vi "proiectu fara drona_with_phone.vi"() -> ()   [LabVIEW 2015]
uses:
  <vilib>/vision/driver/NI_Vision_Acquisition_Software.lvlib
  <vilib>/userdefined/High Color/IMAQdx.ctl
panel:
  out "Grabbing images":bool
  in  "Tab Control":T1(tab)
  in  "Grab picture":bool
  out "Number of photos":i32
  in  "Stop grabbing":bool
  out "Please select your destination":T2(plugin-control)
  out "START LOCATION":T2(plugin-control)
  out "CAR PATH":T2(plugin-control)
  out "Elapsed time":dbl
  out "Color segmentation":bool
  out "Started creating image from matrix":bool
  in  "?":bool
  out "Computing Path for the car":bool
  out "Finding START/STOP":bool
  out "Started stitching":bool
  # "Please wait while the images are processed and stitched together!"
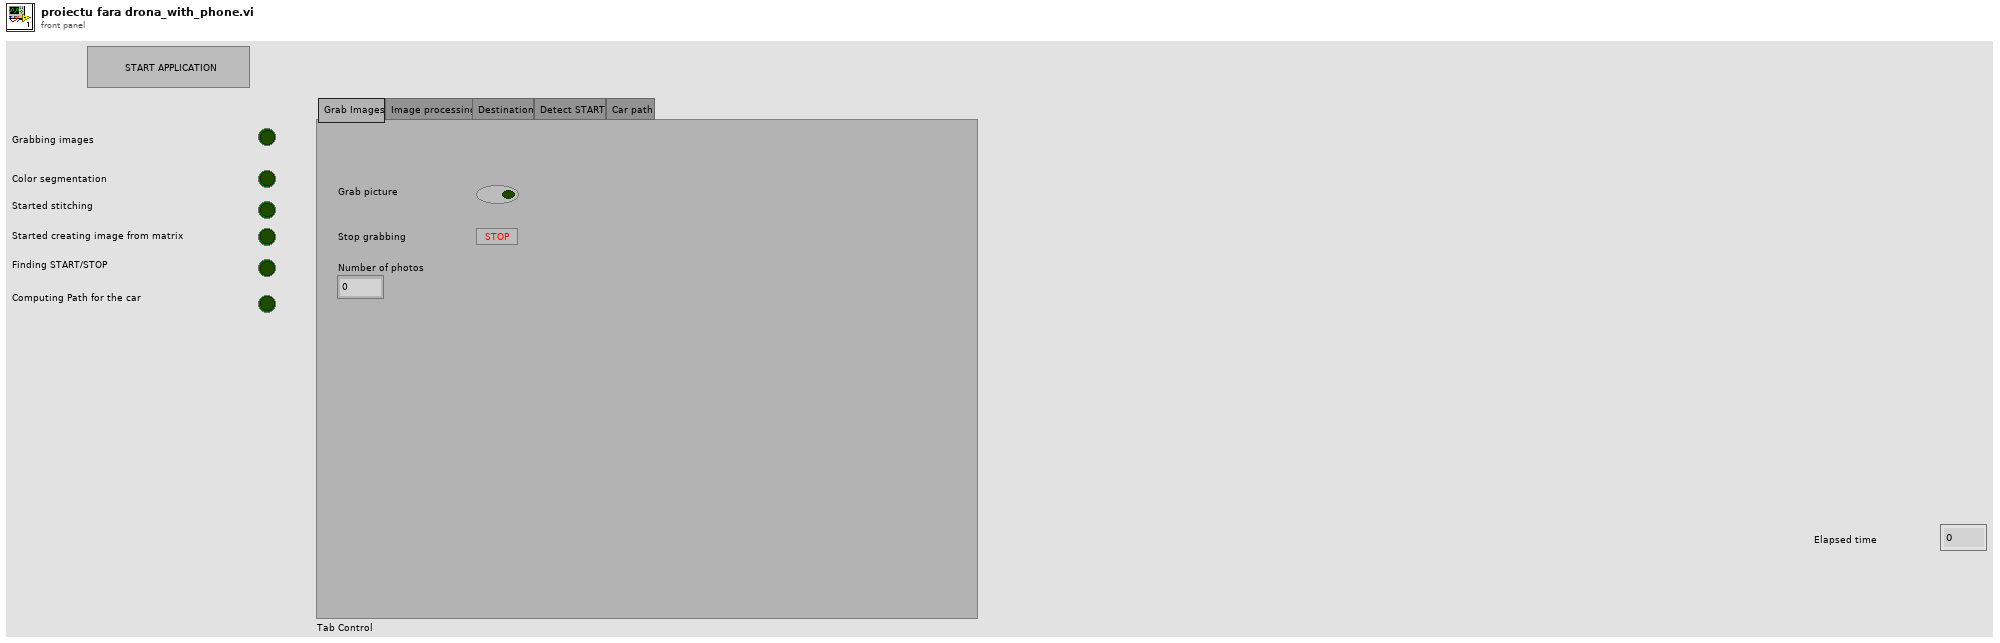
[diagram p1: front panel]
types:
  T1 = enum32{"Grab Images", "Image processing", "Destination", "Detect START", "Car path"}
  T2 = typedef "IMAQ Image.ctl" = refnum<image>
  T3 = typedef "IMAQdx.ctl" = refnum<k21>
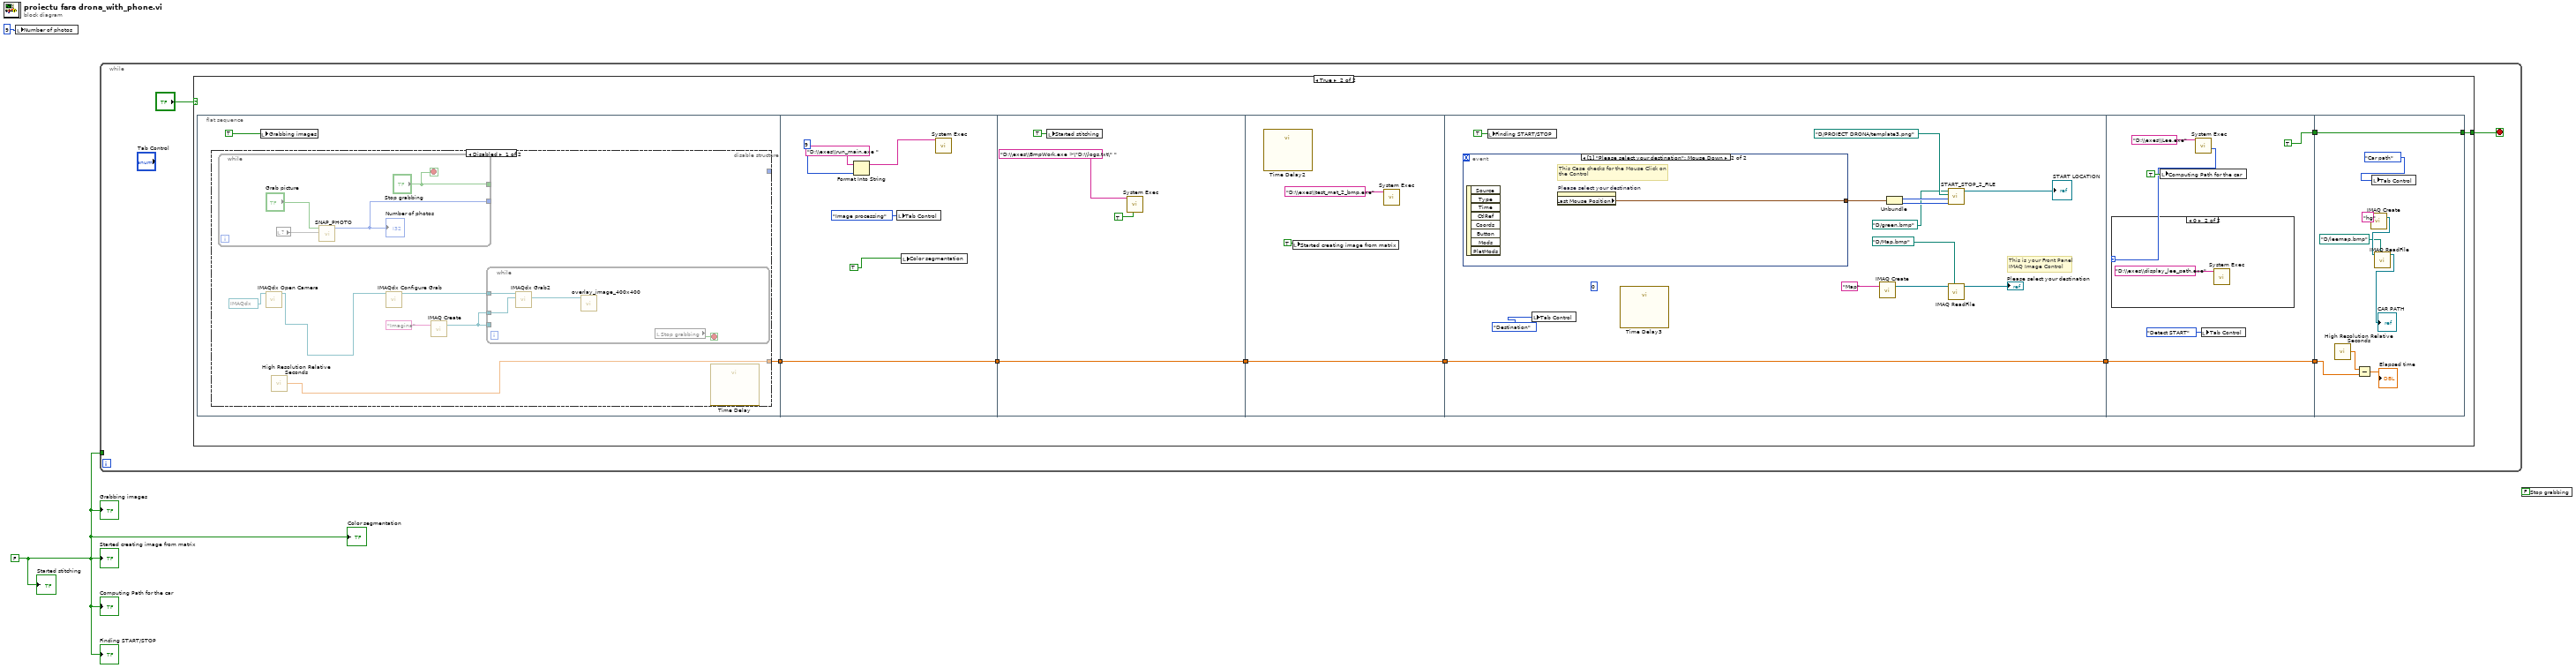
[diagram p0: block diagram]
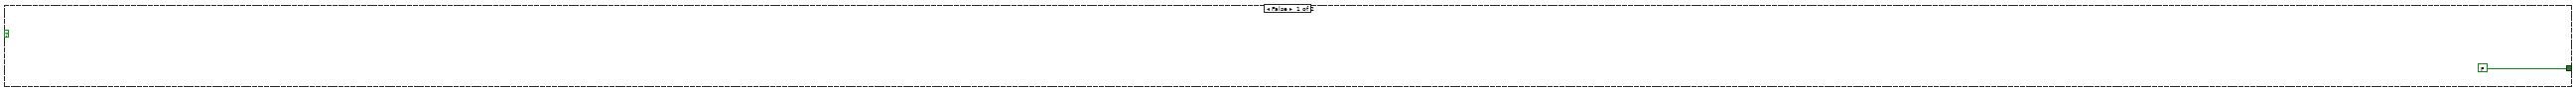
[diagram p2: hidden frame]
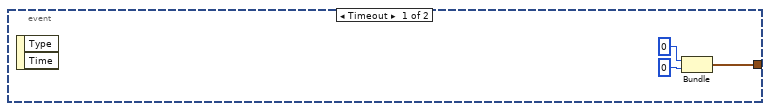
[diagram p4: hidden frame]
diagram:
  w1 = FALSE
  n1 = local write "Number of photos"(9 ("Number of photos")) -> ()
  n2 = while {
    tunnel: w1 -> [_]
    stop <- w4 stop-if-true
    n3 = case shown="True" "?" {
      tunnel: [FALSE w14] -> w4
      frame False {
      }
      frame True {
        n4 = flat-sequence {
          tunnel: [w15] -> w7
          tunnel: [w37] -> w8
          tunnel: w7 -> [w37]
          tunnel: [w40] -> w9
          tunnel: w8 -> [w40]
          tunnel: [w43] -> w10
          tunnel: w9 -> [w43]
          tunnel: [w48] -> w11
          tunnel: w10 -> [w48]
          tunnel: [TRUE] -> w13
          tunnel: [w64] -> w12
          tunnel: w11 -> [w64]
          tunnel: [w78] -> w14
          tunnel: w13 -> [w78]
          tunnel: w12 -> [w71]
          frame #0 {
            n5 = disable-structure shown="Disabled" {
              disable-tunnel: [w18 _] -> w15
              disable-tunnel: _ -> [w17 _]
              frame Disabled {
                n6 = while {
                  tunnel: ["Stop grabbing"] -> _
                  tunnel: [w29] -> _
                  stop <- "Stop grabbing" stop-if-true
                  n7 = local read item#-1() -> (w31)
                  n8 = call "SNAP_PHOTO.vi"("Image"=w31, "Boolean"="Grab picture") -> ("Numeric 2"=w29:i32)  [unwired: 9 in]
                  "Number of photos" <- w29
                }
                n9 = call <vilib>:"IMAQdx Open Camera.vi"("Session In"=T3 "cam2") -> ("Session Out"=w19:T3)  [unwired: 9 in, 1 out]
                n10 = call <vilib>:"High Resolution Relative Seconds.vi"() -> ("relative seconds"=w18:dbl)
                n11 = call <vilib>:"IMAQdx Configure Grab.vi"("Session In"=w19) -> ("Session Out"=w21:T3)  [unwired: 9 in, 1 out]
                n12 = call "IMAQ Create"("Image Name"="Imagina") -> ("New Image"=w22:T2)  [unwired: 4 in, 1 out]
                n13 = while {
                  tunnel: w22 -> [_]
                  tunnel: w22 -> [w28]
                  tunnel: w21 -> [w27]
                  stop <- w26 stop-if-true
                  n14 = call <vilib>:"IMAQdx Grab2.vi"("Image In"=w28, "Session In"=w27) -> ("Image Out"=w25:T2)  [unwired: 6 in, 3 out]
                  n15 = call "overlay_image_400x400.vi"("Image 2"=w25) -> ("Image"=w24:T2)  [unwired: 10 in]
                  n16 = local read "Stop grabbing"() -> (w26:bool)
                }
                n17 = call "Time Delay"() -> ()  [unwired: 11 in, 1 out]
              }
              frame Enabled {
              }
            }
            n18 = local write "Grabbing images"(TRUE) -> ()
          }
          frame #1 {
            n19 = Format Into String(initial string="D:\\exes\\run_main.exe ", 9) -> (resulting string=w35:string)  [unwired: 2 in, 1 out]
            n20 = local write "Tab Control"(T1."Image processing" ("Tab Control")) -> ()
            n21 = local write "Color segmentation"(TRUE) -> ()
            n22 = call <vilib>:"System Exec.vi"("command line"=w35) -> ()  [unwired: 7 in, 4 out]
          }
          frame #2 {
            n23 = local write "Started stitching"(TRUE) -> ()
            n24 = call <vilib>:"System Exec.vi"("run minimized? (F)"=TRUE, "command line"="D:\\exes\\BmpWork.exe >\"D:\\logs.txt\" ") -> ()  [unwired: 6 in, 4 out]
          }
          frame #3 {
            n25 = call "Time Delay2"() -> ()  [unwired: 11 in, 1 out]
            n26 = local write "Started creating image from matrix"(TRUE) -> ()
            n27 = call <vilib>:"System Exec.vi"("command line"="D:\\exes\\test_mat_2_bmp.exe") -> ()  [unwired: 7 in, 4 out]
          }
          frame #4 {
            (unwired) 0 ("index")
            # "This is your Front Panel\nIMAQ Image Control"
            n28 = event shown="[1] \"Please select your destination\": Mouse Down" {
              selector: _ -> [_ _]
              dyn-events: _ -> [_ _]
              timeout: _ -> [_ _]
              tunnel: [w59 w62] -> w49
              event Timeout {
                n29 = event-data() -> ()  [unwired: 3 out]
                n30 = Bundle(0, 0) -> (w59:cluster{i32, i32})  [unwired: 1 in]
              }
              event "Please select your destination": Mouse Down {
                # "This Case checks for the Mouse Click on\nthe Control"
                n31 = event-data() -> ()  [unwired: 9 out]
                n32 = property on="Please select your destination" class="ImageControl"() -> ("Last Mouse Position"=w62:cluster{"X":i32, "Y":i32})  [unwired: 2 in, 2 out]
              }
            }
            n33 = local write "Finding START/STOP"(TRUE) -> ()
            n34 = local write "Tab Control"(T1."Destination" ("Tab Control")) -> ()
            n35 = call "Time Delay3"() -> ()  [unwired: 11 in, 1 out]
            n36 = call "IMAQ Create"("Image Name"="Map") -> ("New Image"=w55:T2)  [unwired: 4 in, 1 out]
            n37 = Unbundle(w49) -> ("X"=w51:i32, "Y"=w50:i32)
            n38 = call "START_STOP_2_FILE.vi"("stop_y"=w50, "stop_x"=w51, "Template"=path "D:/PROIECT DRONA/template3.png" ("Path to template"), "MAP"=path "D:/green.bmp") -> ("Image"=→"START LOCATION":T2)  [unwired: 7 in]
            n39 = call "IMAQ ReadFile"("File Path"=path "D:/Map.bmp" ("Fisierul Text"), "Image"=w55) -> ("Image Out"=→"Please select your destination":T2)  [unwired: 5 in, 4 out]
          }
          frame #5 {
            n40 = local write "Computing Path for the car"(TRUE) -> ()
            n41 = call <vilib>:"System Exec.vi"("command line"="D:\\exes\\Lee.exe") -> ("return code"=w65:i32)  [unwired: 7 in, 3 out]
            n42 = case shown="0" w65 {
              frame Default {
              }
              frame 0 {
                n43 = call <vilib>:"System Exec.vi"("command line"="D:\\exes\\display_lee_path.exe") -> ()  [unwired: 7 in, 4 out]
              }
            }
            n44 = local write "Tab Control"(T1."Detect START" ("Tab Control")) -> ()
          }
          frame #6 {
            n45 = call <vilib>:"High Resolution Relative Seconds.vi"() -> ("relative seconds"=w72:dbl)
            n46 = Subtract(x=w72, y=w71) -> (x-y=→"Elapsed time":dbl)
            n47 = call "IMAQ Create"("Image Name"="hg") -> ("New Image"=w76:T2)  [unwired: 4 in, 1 out]
            n48 = local write "Tab Control"(T1."Car path" ("Tab Control")) -> ()
            n49 = call "IMAQ ReadFile"("File Path"=path "D:/leemap.bmp", "Image"=w76) -> ("Image Out"=→"CAR PATH":T2)  [unwired: 5 in, 4 out]
          }
        }
      }
    }
  }
  n50 = local write "Stop grabbing"(FALSE) -> ()
  "Finding START/STOP" <- w1
  "Computing Path for the car" <- w1
  "Started stitching" <- w1
  "Grabbing images" <- w1
  "Started creating image from matrix" <- w1
  "Color segmentation" <- w1
